vi "BioIsFailed.vi"(3 "ErrorCode":i32) -> (1 "IsFailed?":bool)   [LabVIEW 2020]
doc: "Check whether the error code belongs to fail or warning."
uses:
  AdvLvDaq.dll
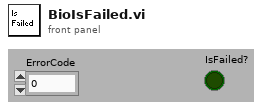
[diagram p1: front panel]
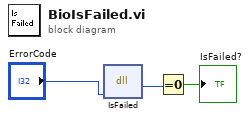
[diagram p0: block diagram]
diagram:
  n1 = dll-call lib="AdvLvDaq.dll" fn="IsFailed"("err"="ErrorCode") -> ("return type"=w2:i32)  [unwired: 4 in, 2 out]
  n2 = Equal To 0?(x=w2) -> (x = 0?=→"IsFailed?":bool)
